vi "CalculateOffset.vi"(8 "SSC":dbl, 9 "Range Std.":dbl, 10 "Range":dbl, 11 "Tube Length":dbl) -> (2 "Raw Offset Value":dbl, 3 "Offset Value":dbl)   [LabVIEW 2018]
uses:
  Analysis/Global Tube Length.vi
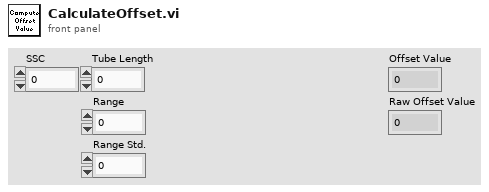
[diagram p1: front panel]
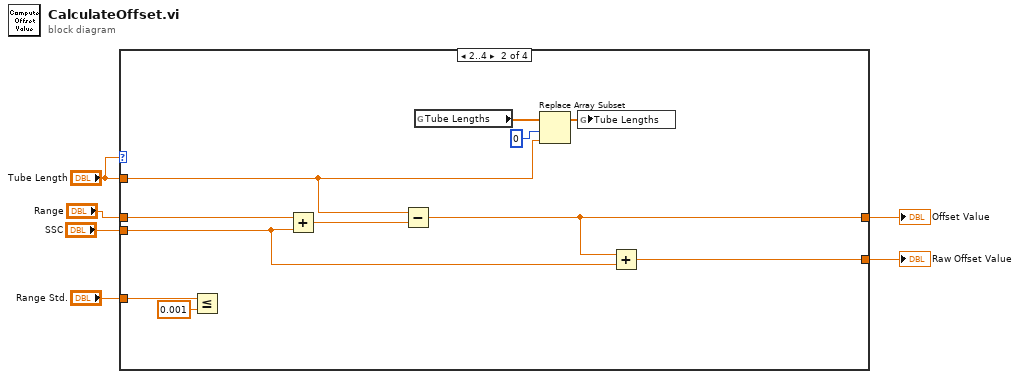
[diagram p0: block diagram]
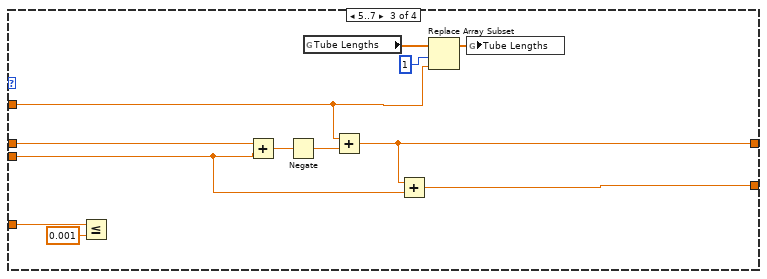
[diagram p3: hidden frame]
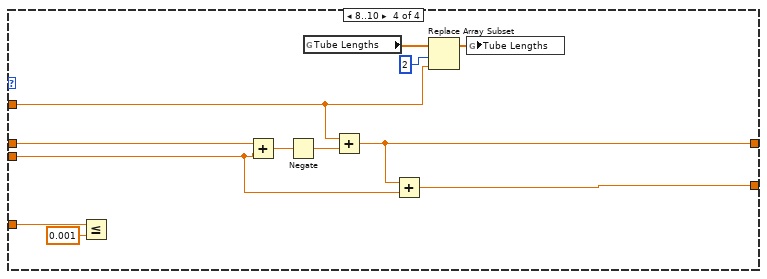
[diagram p4: hidden frame]
diagram:
  n1 = case shown="2..4" "Tube Length" {
    tunnel: "Tube Length" -> [_ w9 w25 w37]
    tunnel: "Range" -> [_ w13 w24 w36]
    tunnel: "Range Std." -> [_ w12 w23 w35]
    tunnel: [_ w7 w20 w32] -> w3
    tunnel: "SSC" -> [_ w11 w19 w31]
    tunnel: [_ w10 w18 w30] -> w1
    frame 0, Default {
    }
    frame 2..4 {
      n2 = Less Or Equal?(x=w12, y=0.001) -> ()  [unwired: 1 out]
      n3 = Add(x=w13, y=w11) -> (x+y=w8:dbl)
      n4 = Subtract(x=w9, y=w8) -> (x-y=w7:dbl)
      n5 = global read "Global Tube Length.vi" "Tube Lengths"() -> (w15:dbl[])
      n6 = Replace Array Subset(array=w15, new element=w9, index=0) -> (w16:dbl[])
      n7 = global write "Global Tube Length.vi" "Tube Lengths"(w16) -> ()
      n8 = Add(x=w7, y=w11) -> (x+y=w10:dbl)
    }
    frame 5..7 {
      n9 = Less Or Equal?(x=w23, y=0.001) -> ()  [unwired: 1 out]
      n10 = Add(x=w24, y=w19) -> (x+y=w22:dbl)
      n11 = Negate(x=w22) -> (-x=w21:dbl)
      n12 = global read "Global Tube Length.vi" "Tube Lengths"() -> (w27:dbl[])
      n13 = Add(x=w25, y=w21) -> (x+y=w20:dbl)
      n14 = Add(x=w20, y=w19) -> (x+y=w18:dbl)
      n15 = Replace Array Subset(array=w27, new element=w25, index=1) -> (w28:dbl[])
      n16 = global write "Global Tube Length.vi" "Tube Lengths"(w28) -> ()
    }
    frame 8..10 {
      n17 = Less Or Equal?(x=w35, y=0.001) -> ()  [unwired: 1 out]
      n18 = Add(x=w36, y=w31) -> (x+y=w34:dbl)
      n19 = Negate(x=w34) -> (-x=w33:dbl)
      n20 = global read "Global Tube Length.vi" "Tube Lengths"() -> (w39:dbl[])
      n21 = Add(x=w37, y=w33) -> (x+y=w32:dbl)
      n22 = Add(x=w32, y=w31) -> (x+y=w30:dbl)
      n23 = Replace Array Subset(array=w39, new element=w37, index=2) -> (w40:dbl[])
      n24 = global write "Global Tube Length.vi" "Tube Lengths"(w40) -> ()
    }
  }
  "Offset Value" <- w3
  "Raw Offset Value" <- w1
